vi "Init UI.vi"(8 "error in (no error)":errorcluster, 11 "Channel in":refnum<class "Channel.lvclass">) -> (0 "error out":errorcluster, 3 "Channel out":refnum<class "Channel.lvclass">)   [LabVIEW 2019, in "Channel.lvclass"]
uses:
  Channel.lvclass
  Packed Libraries/Messaging.lvlibp
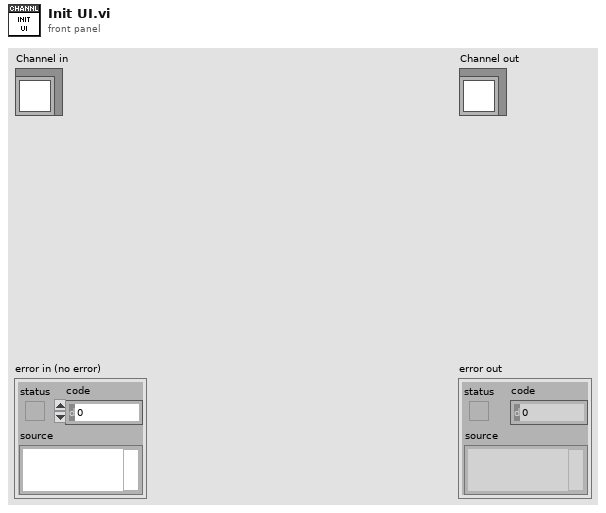
[diagram p1: front panel]
types:
  T1 = typedef "Audio Processing.lvlibp/Value Properties.ctl" = cluster{"Lower":dbl, "Upper":dbl, "Default":dbl, "Increment":dbl}
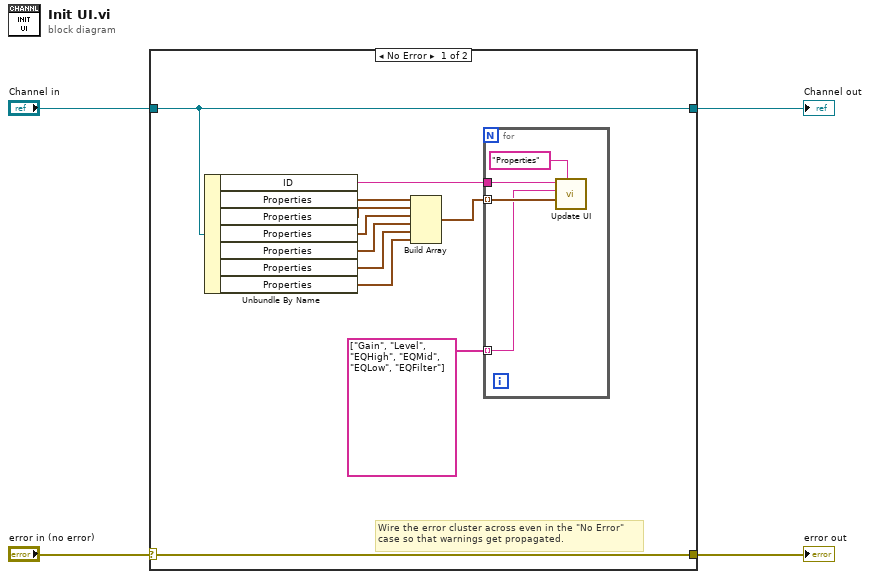
[diagram p0: block diagram]
diagram:
  n1 = case shown="No Error" "error in (no error)" {
    selector: "error in (no error)" -> [w15 w21]
    tunnel: [w15 w21] -> w2
    tunnel: [w14 w20] -> w1
    tunnel: "Channel in" -> [w14 w20]
    frame No Error {
      # "Wire the error cluster across even in the \"No Error\"\ncase so that warnings get propagated."
      n2 = Unbundle By Name(w14) -> ("ID"=w13:string, "Properties"=w12:T1, "Properties"=w9:T1, "Properties"=w8:T1, "Properties"=w7:T1, "Properties"=w6:T1, "Properties"=w5:T1)
      n3 = Build Array(w12, w9, w8, w7, w6, w5) -> (w11:T1[])
      n4 = for {
        tunnel: w13 -> [w19]
        tunnel: w11 -> [w18] mode=indexing
        tunnel: string[] ["Gain", "Level", "EQHigh", "EQMid", "EQLow", "EQFilter"] -> [w17] mode=indexing
        n5 = call "Update UI.vi"("Message (Value Change)"="Properties", "Data"=w18, "Target"=w17, "ID"=w19) -> ()  [unwired: 7 in, 1 out]
      }
    }
    frame Error {
    }
  }
  "error out" <- w2
  "Channel out" <- w1
